vi "Position Virtual Joystick.vi"(8 "error in (no error)":errorcluster, 11 "Joystick Refnum":refnum<vi>) -> (0 "error out":errorcluster)   [LabVIEW 2014]
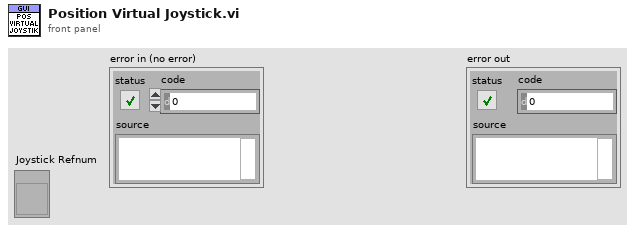
[diagram p1: front panel]
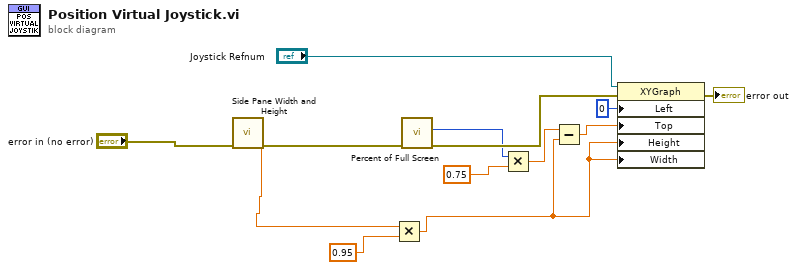
[diagram p0: block diagram]
diagram:
  n1 = call "Side Pane Width and Height.vi"("error in (no error)"="error in (no error)") -> ("error out"=w12:errorcluster, "Width"=w3:dbl)  [unwired: 8 in, 1 out]
  n2 = Multiply(x=w3, y=0.95) -> (x*y=w1:dbl)
  n3 = call "Percent of Full Screen.vi"("error in (no error)"=w12) -> ("error out"=w11:errorcluster, "Bottom"=w6:i16)  [unwired: 8 in, 1 out]
  n4 = Multiply(x=w6, y=0.75) -> (x*y=w4:dbl)
  n5 = Subtract(x=w4, y=w1) -> (x-y=w9:dbl)
  n6 = property class="XYGraph"(reference="Joystick Refnum", error in=w11, "Left"=0 ("Position:Left"), "Top"=w9, "Height"=w1, "Width"=w1) -> (error out=→"error out":errorcluster)  [unwired: 1 out]
